vi "ArrayDemo.vi"() -> ()   [LabVIEW 2019]
panel:
  out "Array Size":dbl
  out "Minimum Value":dbl
  out "Minimum Value Index":dbl
  out "Maximum Value Index":dbl
  out "Maximum Value":dbl
  in  "?":bool
  in  "OK Button":bool
  in  "Maximum Value":dbl=100.0
  in  "Minimum Value":dbl
  in  "Number of Array Elements":dbl=1000.0
  out "Array":dbl[](array[numeric])
  # "Integers Only"
  # "Real Numbers"
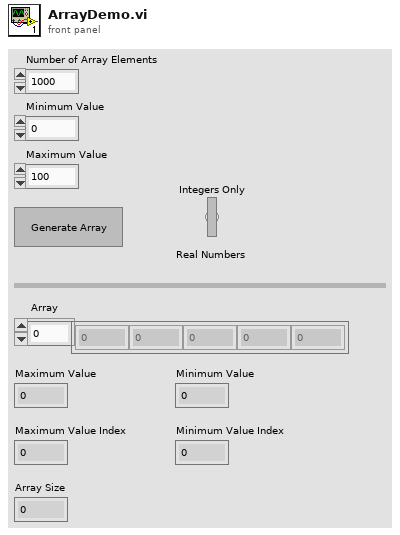
[diagram p1: front panel]
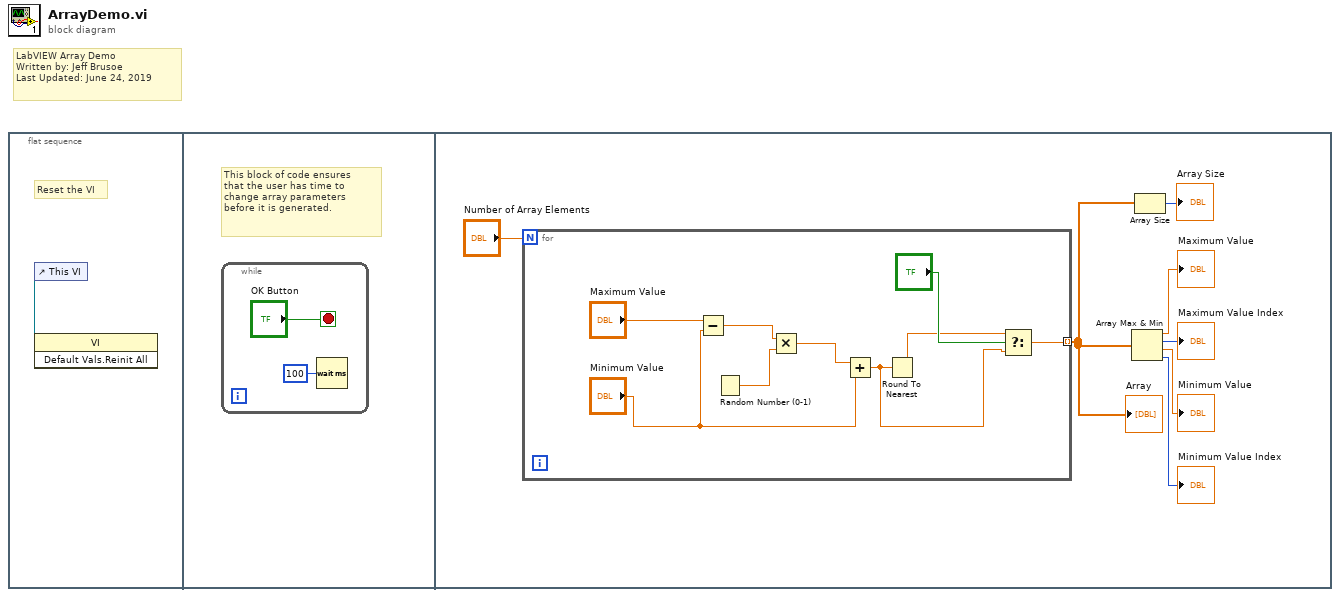
[diagram p0: block diagram]
diagram:
  # "LabVIEW Array Demo\nWritten by: Jeff Brusoe\nLast Updated: June 24, 2019"
  n1 = flat-sequence {
    frame #0 {
      # "Reset the VI"
      n2 = control-ref of="This VI"() -> (w1:refnum<vi>)
      n3 = invoke class="VI" method="Default Vals.Reinit All"(reference=w1) -> ()  [unwired: 2 in, 3 out]
    }
    frame #1 {
      # "This block of code ensures\nthat the user has time to \nchange array parameters\nbefore it is generated."
      n4 = while {
        stop <- "OK Button" stop-if-true
        n5 = Wait (ms)(milliseconds to wait=u32 100) -> ()  [unwired: 1 out]
      }
    }
    frame #2 {
      n6 = for {
        N: "Number of Array Elements" -> [_]
        tunnel: [w11] -> w4 mode=indexing
        n7 = Subtract(x="Maximum Value", y="Minimum Value") -> (x-y=w15:dbl)
        n8 = Random Number (0-1)() -> (number: 0 to 1=w18:dbl)
        n9 = Multiply(x=w15, y=w18) -> (x*y=w17:dbl)
        n10 = Add(x=w17, y="Minimum Value") -> (x+y=w12:dbl)
        n11 = Round To Nearest(number=w12) -> (nearest integer value=w13:dbl)
        n12 = Select(t=w13, s="?", f=w12) -> (s? t:f=w11:dbl)
      }
      "Array" <- w4
      n13 = Array Max & Min(array=w4) -> (max value=→"Maximum Value":dbl, max index (indices)=→"Maximum Value Index":i32, min value=→"Minimum Value":dbl, min index (indices)=→"Minimum Value Index":i32)
      n14 = Array Size(array=w4) -> (size(s)=→"Array Size":i32)
    }
  }
